vi "Hysteresis-GetPreCorrectedImage.vi"(4 "fwd?":bool=TRUE, 6 "frame up?":bool=TRUE, 7 "pixel to delete":i32, 8 "Polynomial Coefficients bwd":dbl[](array[numeric]), 9 "Relative Range":dbl format="%#_13g", 10 "Polynomial Coefficients fwd":dbl[](array[numeric]), 11 "Before Correction Data":dbl[][](array[numeric])) -> (3 "After Correction data":dbl[][](array[numeric]))   [LabVIEW 2016]
panel:
  out "After Correction":dbl[][](graph)
  out "Before Correction":dbl[][](graph)
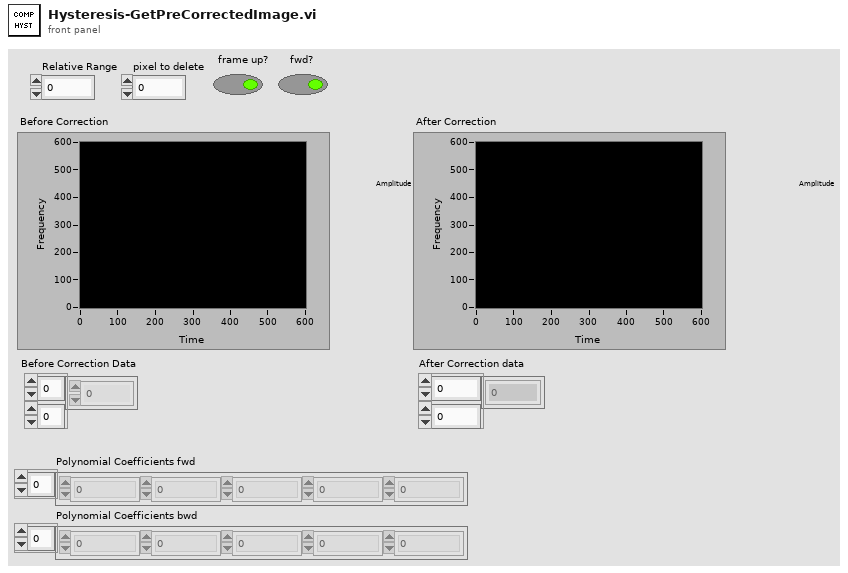
[diagram p1: front panel]
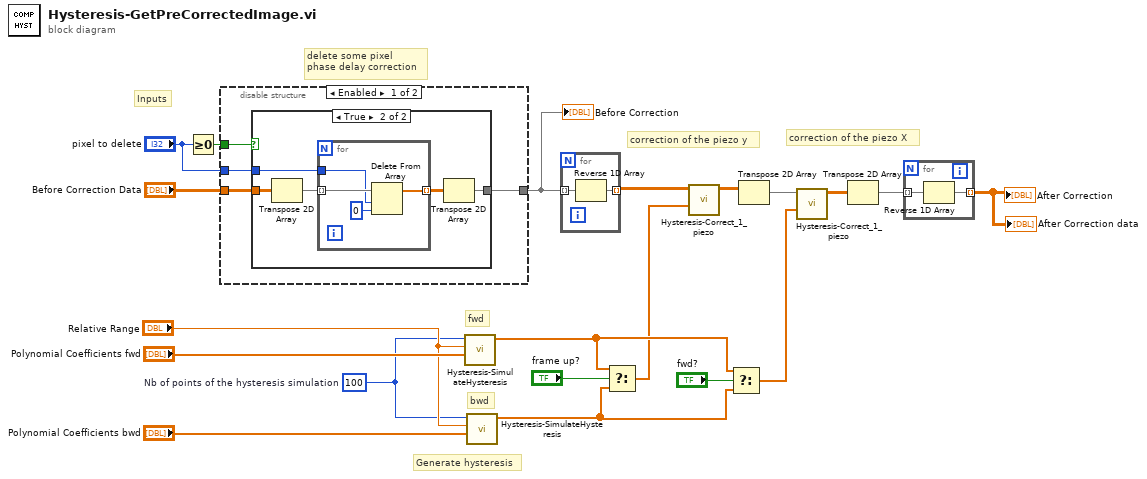
[diagram p0: block diagram]
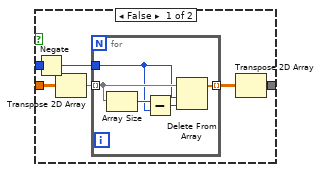
[diagram p2: hidden frame]
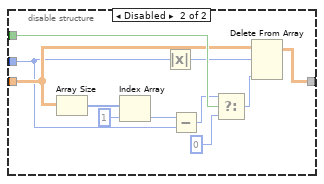
[diagram p3: hidden frame]
diagram:
  w10 = 100  # Nb of points of the hysteresis simulation
  # "Generate hysteresis"
  # "bwd"
  # "correction of the piezo y"
  # "correction of the piezo X"
  # "Inputs"
  # "fwd"
  # "delete some pixel\nphase delay correction"
  n1 = Greater Or Equal To 0?(x="pixel to delete") -> (x >= 0?=w16:bool)
  n2 = disable-structure shown="Enabled" {
    disable-tunnel: w16 -> [w24 w55]
    disable-tunnel: "pixel to delete" -> [w23 w46]
    disable-tunnel: "Before Correction Data" -> [w22 w47]
    disable-tunnel: [w21 w52] -> w7
    frame Enabled {
      n3 = case shown="True" w24 {
        tunnel: w23 -> [w29 w36]
        tunnel: w22 -> [w30 w37]
        tunnel: [w25 w38] -> w21
        frame False {
          n4 = Negate(x=w29) -> (-x=w28:i32)
          n5 = Transpose 2D Array(2D array=w30) -> (transposed array=w26:dbl[][])
          n6 = for {
            tunnel: w26 -> [w34] mode=indexing
            tunnel: [w35] -> w27 mode=indexing
            tunnel: w28 -> [w32]
            n7 = Array Size(array=w34) -> (size(s)=w33:i32)
            n8 = Subtract(x=w33, y=w32) -> (x-y=w31:i32)
            n9 = Delete From Array(array=w34, length=w32, index=w31) -> (array with subset deleted=w35:dbl[])  [unwired: 1 out]
          }
          n10 = Transpose 2D Array(2D array=w27) -> (transposed array=w25:dbl[][])
        }
        frame True {
          n11 = Transpose 2D Array(2D array=w37) -> (transposed array=w40:dbl[][])
          n12 = for {
            tunnel: w40 -> [w44] mode=indexing
            tunnel: [w43] -> w39 mode=indexing
            tunnel: w36 -> [w42]
            n13 = Delete From Array(array=w44, length=w42, index=0) -> (array with subset deleted=w43:dbl[])  [unwired: 1 out]
          }
          n14 = Transpose 2D Array(2D array=w39) -> (transposed array=w38:dbl[][])
        }
      }
    }
    frame Disabled {
      n15 = Array Size(array=w47) -> (size(s)=w51:i32[])
      n16 = Index Array(array=w51, index=1) -> (element=w49:i32)
      n17 = Absolute Value(x=w46) -> (abs(x)=w45:i32)
      n18 = Subtract(x=w49, y=w46) -> (x-y=w54:i32)
      n19 = Select(t=w54, s=w55, f=0) -> (s? t:f=w53:i32)
      n20 = Delete From Array(array=w47, length=w45, index (col)=w53) -> (array with subset deleted=w52:dbl[][])  [unwired: 1 in, 1 out]
    }
  }
  "Before Correction" <- w7
  n21 = call "Hysteresis-SimulateHysteresis.vi"("Polynomial Coefficients"="Polynomial Coefficients fwd", "Relative Range"="Relative Range", "NbPoints"=w10) -> ("Hyst curve"=w9:dbl[])  [unwired: 8 in]
  n22 = call "Hysteresis-SimulateHysteresis.vi"("Polynomial Coefficients"="Polynomial Coefficients bwd", "Relative Range"="Relative Range", "NbPoints"=w10) -> ("Hyst curve"=w17:dbl[])  [unwired: 8 in]
  n23 = for {
    tunnel: [w57] -> w5 mode=indexing
    tunnel: w7 -> [w56] mode=indexing
    n24 = Reverse 1D Array(array=w56) -> (reversed array=w57:dbl[])
  }
  n25 = Select(t=w9, s="frame up?", f=w17) -> (s? t:f=w8:dbl[])
  n26 = call "Hysteresis-Correct_1_piezo.vi"("Hyst curve"=w8, "Image In"=w5) -> ("Image Out"=w4:dbl[][])  [unwired: 9 in]
  n27 = Select(t=w9, s="fwd?", f=w17) -> (s? t:f=w19:dbl[])
  n28 = Transpose 2D Array(2D array=w4) -> (transposed array=w3:dbl[][])
  n29 = call "Hysteresis-Correct_1_piezo.vi"("Hyst curve"=w19, "Image In"=w3) -> ("Image Out"=w2:dbl[][])  [unwired: 9 in]
  n30 = Transpose 2D Array(2D array=w2) -> (transposed array=w1:dbl[][])
  n31 = for {
    tunnel: w1 -> [w59] mode=indexing
    tunnel: [w58] -> w6 mode=indexing
    n32 = Reverse 1D Array(array=w59) -> (reversed array=w58:dbl[])
  }
  "After Correction data" <- w6
  "After Correction" <- w6
